vi "2048.vi"() -> ()   [LabVIEW 2013]
panel:
  out "分数":i64=3
  in  "清空按钮":bool
  in  "按钮（退出程序）":bool
  out "错误输出":errorcluster
  in  "错误输入":errorcluster caption="错误输入（无错误）"
  out "2048":u16[][](array[ring])
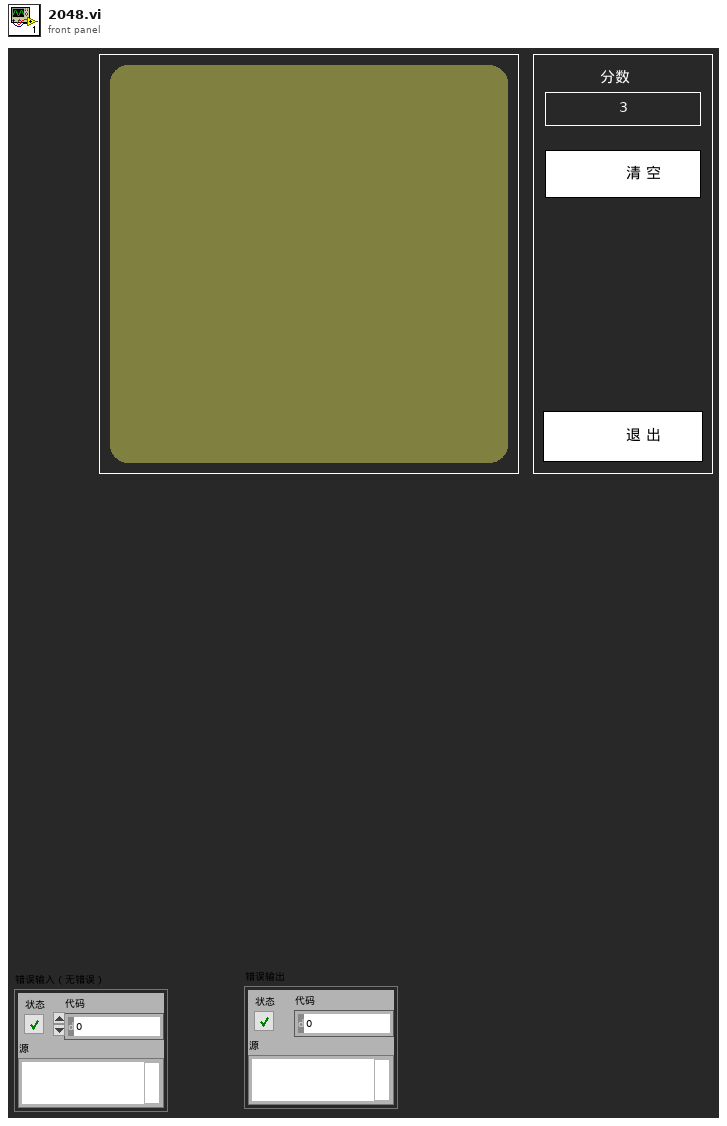
[diagram p1: front panel]
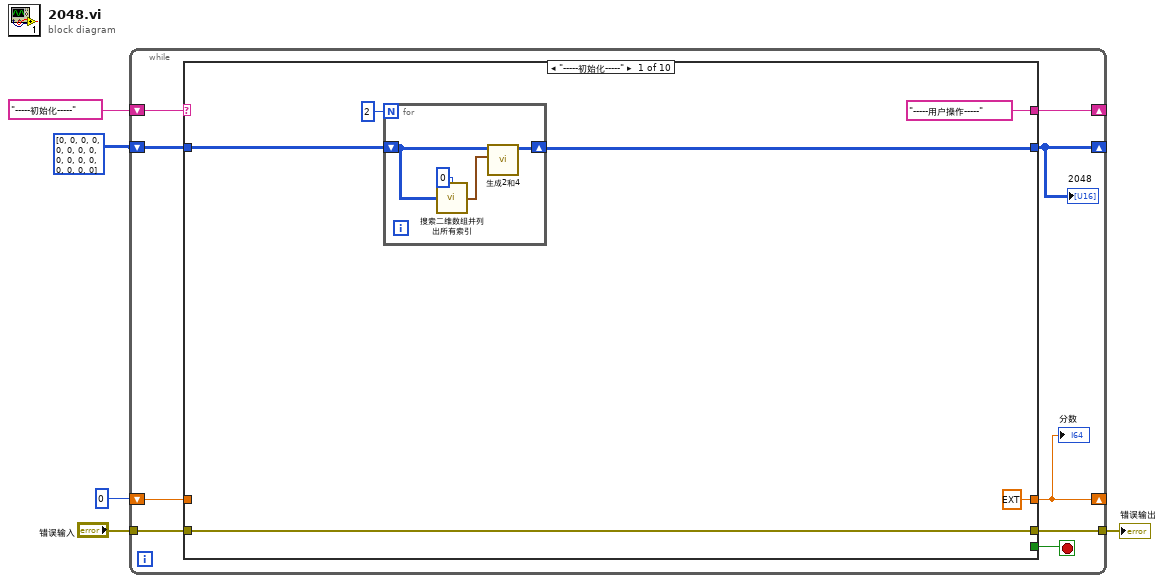
[diagram p0: block diagram]
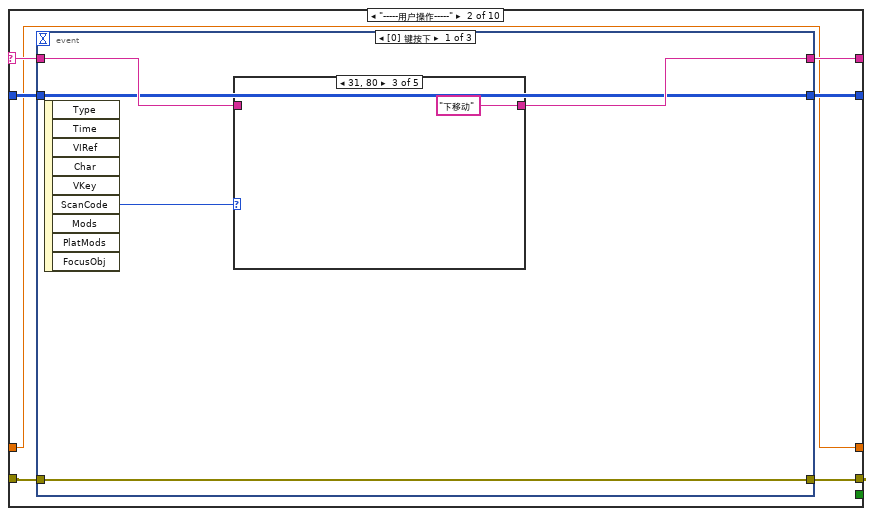
[diagram p2: hidden frame]
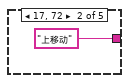
[diagram p4: hidden frame]
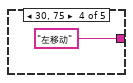
[diagram p5: hidden frame]
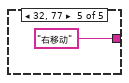
[diagram p6: hidden frame]
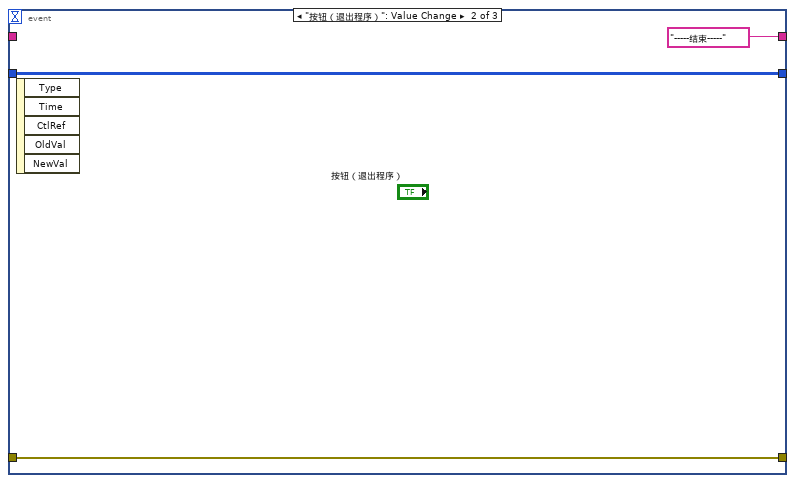
[diagram p7: hidden frame]
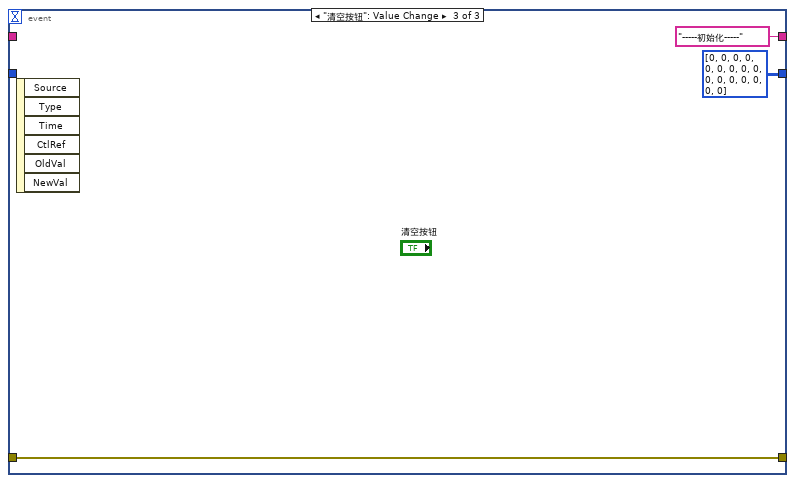
[diagram p8: hidden frame]
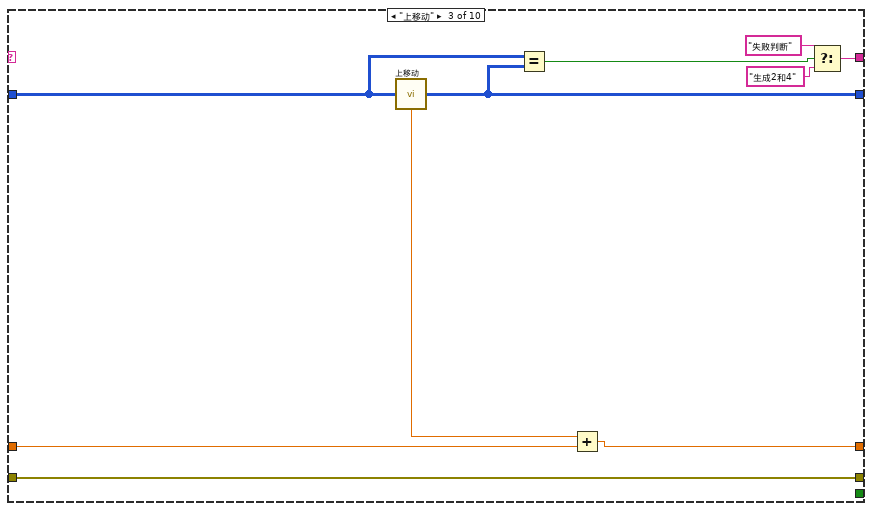
[diagram p9: hidden frame]
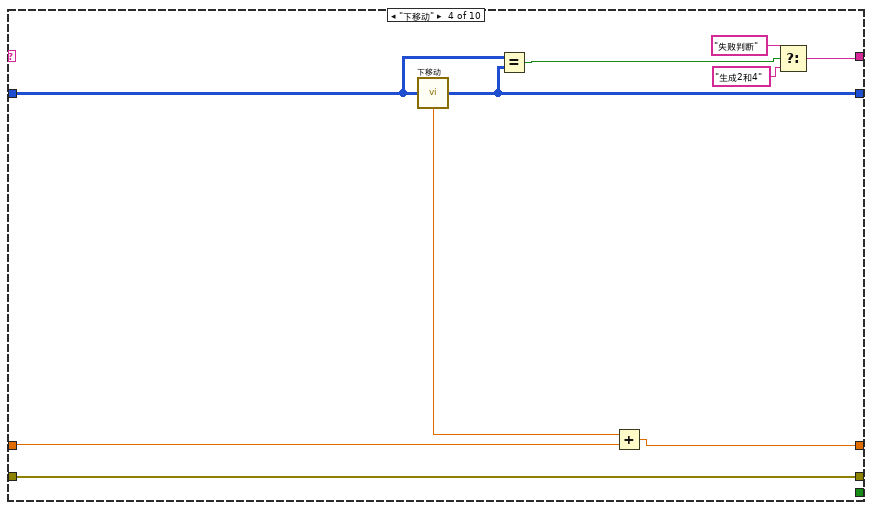
[diagram p10: hidden frame]
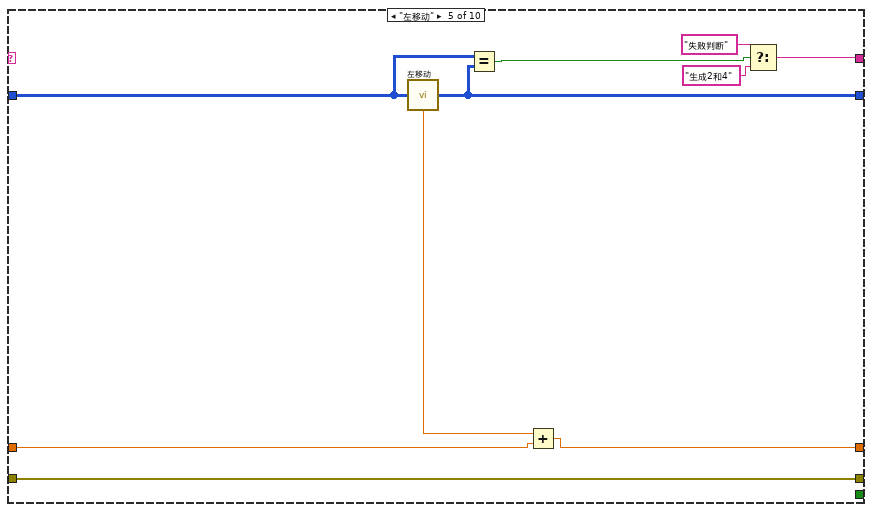
[diagram p11: hidden frame]
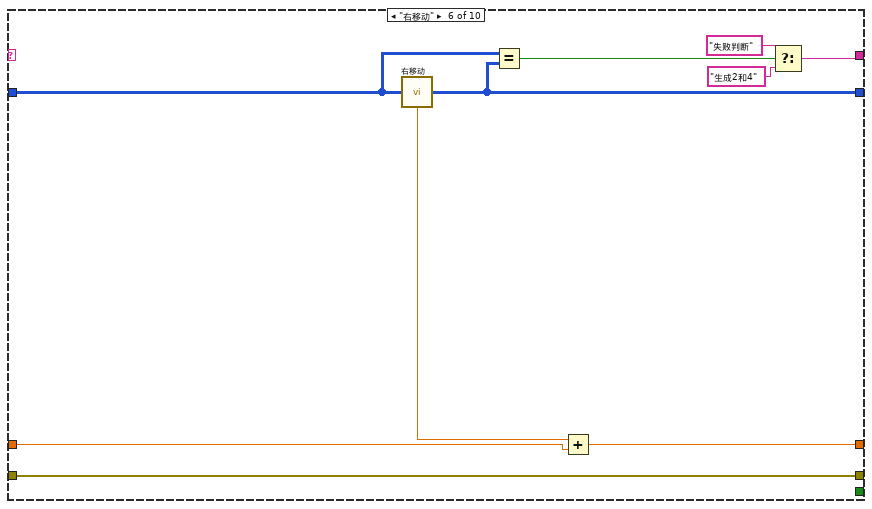
[diagram p12: hidden frame]
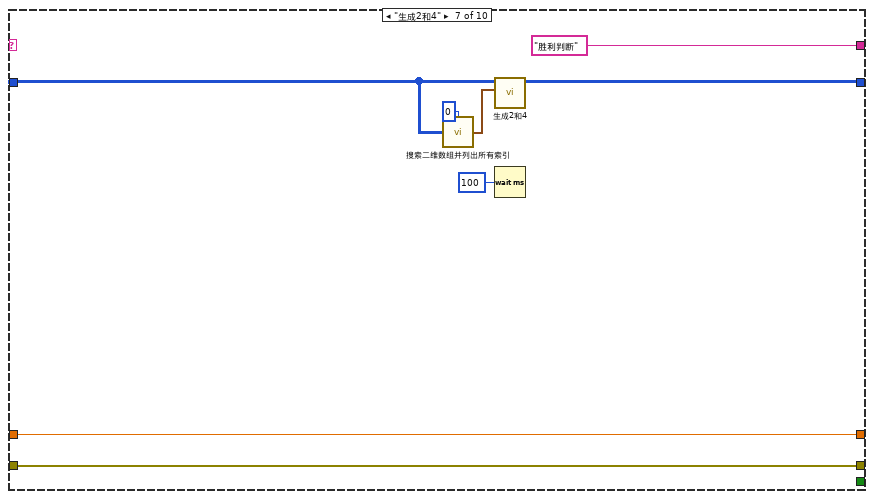
[diagram p13: hidden frame]
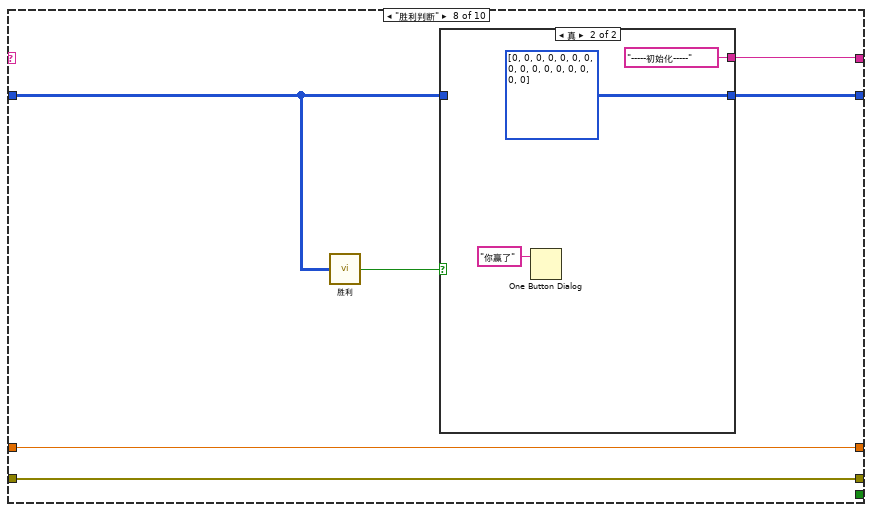
[diagram p14: hidden frame]
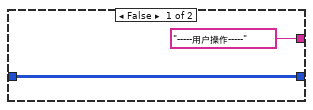
[diagram p15: hidden frame]
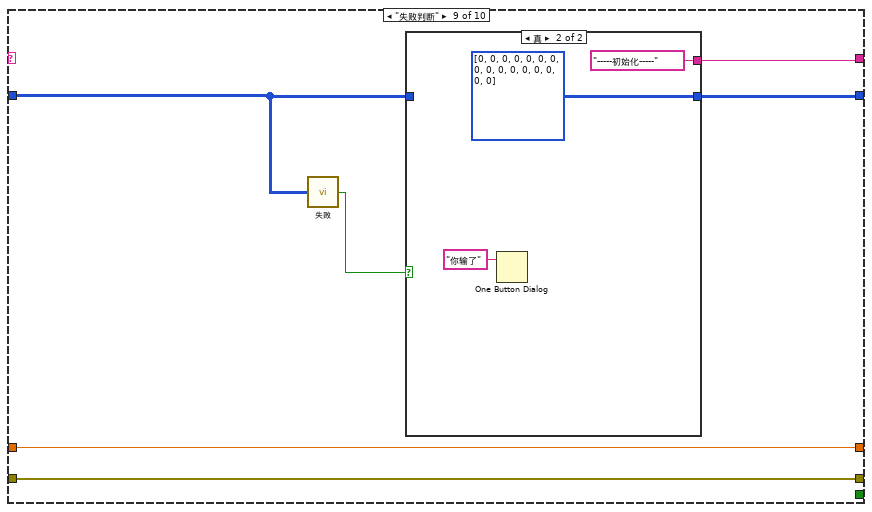
[diagram p16: hidden frame]
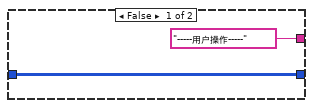
[diagram p17: hidden frame]
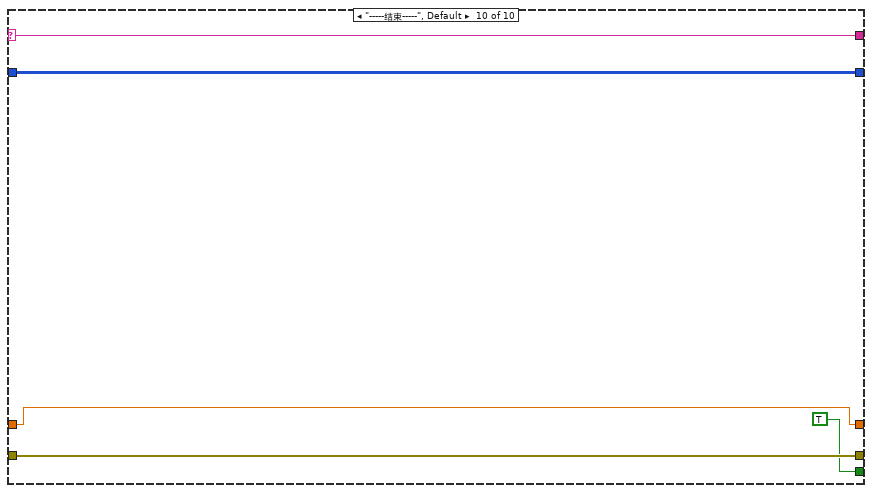
[diagram p18: hidden frame]
diagram:
  n1 = while {
    shift-right: [w11] -> _
    shift-left: "-----初始化-----" -> [w12]
    tunnel: [w14] -> w4
    tunnel: "错误输入" -> [w13]
    shift-right: [w8] -> _
    shift-left: i32[][] [[0, 0, 0, 0], [0, 0, 0, 0], [0, 0, 0, 0], [0, 0, 0, 0]] ("2048") -> [w9]
    shift-right: [w6] -> _
    shift-left: 0 -> [w7]
    stop <- w10 stop-if-true
    n2 = case shown="\"-----初始化-----\"" w12 {
      selector: w12 -> [_ w28 _ _ _ _ _ _ _ w122]
      tunnel: [w20 w31 w57 w67 w77 w87 w95 w101 w112 w121] -> w14
      tunnel: w13 -> [w20 w30 w57 w67 w77 w87 w95 w101 w112 w121]
      tunnel: ["-----用户操作-----" w29 w54 w63 w73 w83 "胜利判断" w97 w111 w122] -> w11
      tunnel: [_ _ _ _ _ _ _ _ _ TRUE] -> w10
      tunnel: [w17 w27 w52 w62 w72 w82 w92 w99 w110 w119] -> w8
      tunnel: w9 -> [w18 w26 w53 w61 w71 w81 w91 w98 w109 w119]
      tunnel: w7 -> [_ w25 w49 w59 w69 w79 w88 w96 w107 w118]
      tunnel: [ext 0.0 w25 w48 w60 w68 w80 w88 w96 w107 w118] -> w6
      frame "-----初始化-----" {
        n3 = for {
          N: 2 -> [_]
          shift-right: [w21] -> w17
          shift-left: w18 -> [w23]
          n4 = call "搜索二维数组并列出所有索引.vi"("搜索值"=0, "数组"=w23) -> ("索引数组"=w22:cluster{i32, i32}[])  [unwired: 2 in]
          n5 = call "生成2和4.vi"("索引数组"=w22, "2048输入"=w23) -> ("2048输出"=w21:i32[][])  [unwired: 9 in]
        }
      }
      frame "-----用户操作-----" {
        n6 = event shown="[0] 键按下" {
          selector: _ -> [_ _ _]
          dyn-events: _ -> [_ _ _]
          timeout: _ -> [_ _ _]
          tunnel: [w36 w44 w47] -> w31
          tunnel: w30 -> [w36 w44 w47]
          tunnel: [w35 "-----结束-----" "-----初始化-----"] -> w29
          tunnel: w28 -> [w34 _ _]
          tunnel: [w32 w42 i32[][] [[0, 0, 0, 0], [0, 0, 0, 0], [0, 0, 0, 0], [0, 0, 0, 0]] ("2048")] -> w27
          tunnel: w26 -> [w32 w42 _]
          event Key Down {
            n7 = event-data() -> ("ScanCode"=w33:i16)  [unwired: 1 in, 8 out]
            n8 = case shown="31, 80" w33 {
              tunnel: [w37 "上移动" "下移动" "左移动" "右移动"] -> w35
              tunnel: w34 -> [w37 _ _ _ _]
              frame 0, Default {
              }
              frame 17, 72 {
              }
              frame 31, 80 {
              }
              frame 30, 75 {
              }
              frame 32, 77 {
              }
            }
          }
          event "按钮（退出程序）": Value Change {
            n9 = event-data() -> ()  [unwired: 1 in, 5 out]
          }
          event "清空按钮": Value Change {
            n10 = event-data() -> ()  [unwired: 1 in, 6 out]
          }
        }
      }
      frame "上移动" {
        n11 = call "上移动.vi"("移动前"=w53) -> ("移动后"=w52:i32[][], "分数"=w50:ext)  [unwired: 2 in]
        n12 = Equal?(x=w53, y=w52) -> (x = y?=w51:bool)
        n13 = Add(x=w50, y=w49) -> (x+y=w48:ext)
        n14 = Select(t="失败判断", s=w51, f="生成2和4") -> (s? t:f=w54:string)
      }
      frame "下移动" {
        n15 = call "下移动.vi"("移动前"=w61) -> ("移动后"=w62:i32[][], "分数"=w58:ext)  [unwired: 2 in]
        n16 = Equal?(x=w61, y=w62) -> (x = y?=w64:bool)
        n17 = Add(x=w58, y=w59) -> (x+y=w60:ext)
        n18 = Select(t="失败判断", s=w64, f="生成2和4") -> (s? t:f=w63:string)
      }
      frame "左移动" {
        n19 = call "左移动.vi"("移动前"=w71) -> ("移动后"=w72:i32[][], "分数"=w70:ext)  [unwired: 2 in]
        n20 = Equal?(x=w71, y=w72) -> (x = y?=w74:bool)
        n21 = Add(x=w70, y=w69) -> (x+y=w68:ext)
        n22 = Select(t="失败判断", s=w74, f="生成2和4") -> (s? t:f=w73:string)
      }
      frame "右移动" {
        n23 = call "右移动.vi"("移动前"=w81) -> ("移动后"=w82:i32[][], "分数"=w78:ext)  [unwired: 2 in]
        n24 = Equal?(x=w81, y=w82) -> (x = y?=w84:bool)
        n25 = Add(x=w78, y=w79) -> (x+y=w80:ext)
        n26 = Select(t="失败判断", s=w84, f="生成2和4") -> (s? t:f=w83:string)
      }
      frame "生成2和4" {
        n27 = call "搜索二维数组并列出所有索引.vi"("搜索值"=0, "数组"=w91) -> ("索引数组"=w94:cluster{i32, i32}[])  [unwired: 2 in]
        n28 = call "生成2和4.vi"("索引数组"=w94, "2048输入"=w91) -> ("2048输出"=w92:i32[][])  [unwired: 9 in]
        n29 = Wait (ms)(milliseconds to wait=u32 100 ("等待时间（毫秒）")) -> ()  [unwired: 1 out]
      }
      frame "胜利判断" {
        n30 = call "胜利.vi"("移动前"=w98) -> ("胜利？"=w100:bool)
        n31 = case shown="真" w100 {
          tunnel: [w103 i32[][] [[0, 0, 0, 0], [0, 0, 0, 0], [0, 0, 0, 0], [0, 0, 0, 0]] ("2048")] -> w99
          tunnel: w98 -> [w103 _]
          tunnel: ["-----用户操作-----" "-----初始化-----"] -> w97
          frame False {
          }
          frame True {
            n32 = One Button Dialog(message="你赢了" ("消息")) -> ()  [unwired: 1 in, 1 out]
          }
        }
      }
      frame "失败判断" {
        n33 = call "失败.vi"("移动前"=w109) -> ("失败？"=w108:bool)
        n34 = case shown="真" w108 {
          tunnel: ["-----用户操作-----" "-----初始化-----"] -> w111
          tunnel: [w113 i32[][] [[0, 0, 0, 0], [0, 0, 0, 0], [0, 0, 0, 0], [0, 0, 0, 0]] ("2048")] -> w110
          tunnel: w109 -> [w113 _]
          frame False {
          }
          frame True {
            n35 = One Button Dialog(message="你输了" ("消息")) -> ()  [unwired: 1 in, 1 out]
          }
        }
      }
      frame "-----结束-----", Default {
      }
    }
    "2048" <- w8
    "分数" <- w6
  }
  "错误输出" <- w4
